vi "Edit Color List Dialog.vi"(10 "Color List":u32[](array[colorbox])=[16777225, 16448250, 16448250, 16448250, 16448250, 16448250, 16448250, 16448250, 16448250, 16448250], 11 "Color List Name":string) -> (0 "OK?":bool, 2 "Color List (out)":u32[](array[colorbox]), 3 "Color List Name (out)":string)   [LabVIEW 2019]
panel:
  in  "Cancel":bool
  in  "OK":bool
  out "# Colors":i32
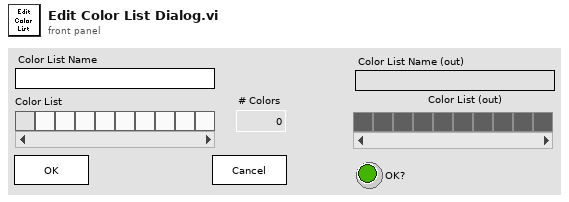
[diagram p1: front panel]
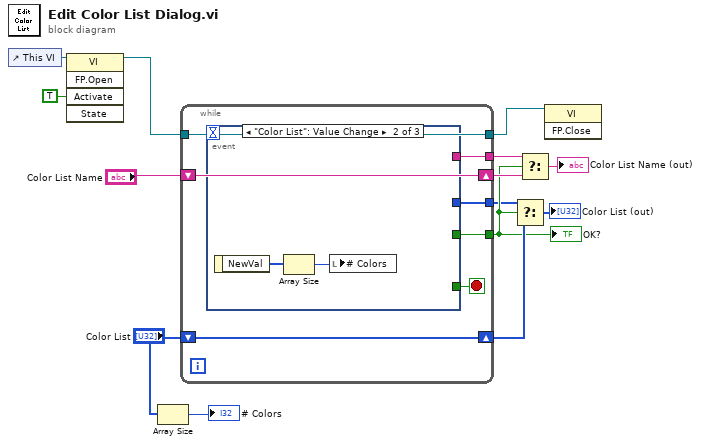
[diagram p0: block diagram]
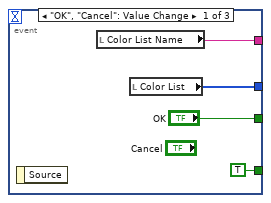
[diagram p2: hidden frame]
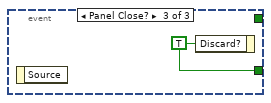
[diagram p3: hidden frame]
diagram:
  n1 = control-ref of="This VI"() -> (w14:refnum<vi>)
  n2 = invoke class="VI" method="FP.Open"(reference=w14, "Activate"=TRUE ("Activate?")) -> (reference out=w8:refnum<vi>)  [unwired: 3 in, 4 out]
  n3 = Array Size(array="Color List") -> (size(s)=→"# Colors":i32)
  n4 = while {
    tunnel: [w20] -> w3
    tunnel: w8 -> [w19]
    tunnel: [w19] -> w13
    shift-right: [w18] -> w12
    shift-left: "Color List" -> [w18]
    shift-right: [w17] -> w5
    shift-left: "Color List Name" -> [w17]
    tunnel: [w16] -> w2
    tunnel: [w15] -> w1
    stop <- w21 stop-if-true
    n5 = event shown="[1] \"Color List\": Value Change" {
      selector: _ -> [_ _ _]
      dyn-events: _ -> [_ _ _]
      timeout: _ -> [_ _ _]
      tunnel: [TRUE ("Discard?") _ w28] -> w21
      tunnel: ["OK" _ _] -> w20
      tunnel: [w23 _ _] -> w16
      tunnel: [w22 _ _] -> w15
      event "OK", "Cancel": Value Change {
        n6 = event-data() -> ()  [unwired: 1 in, 1 out]
        n7 = local read "Color List Name"() -> (w22:string)
        n8 = local read "Color List"() -> (w23:u32[])
      }
      event "Color List": Value Change {
        n9 = event-data() -> ("NewVal"=w27:u32[])  [unwired: 1 in]
        n10 = Array Size(array=w27) -> (size(s)=w26:i32)
        n11 = local write "# Colors"(w26) -> ()
      }
      event Panel Close? {
        w28 = TRUE ("Discard?")
        n12 = event-data() -> ()  [unwired: 1 in, 1 out]
        n13 = event-data("Discard?"=w28) -> ()  [unwired: 1 in, 1 out]
      }
    }
  }
  "OK?" <- w3
  n14 = Select(t=w2, s=w3, f=w12) -> (s? t:f=→"Color List (out)":u32[])
  n15 = Select(t=w1, s=w3, f=w5) -> (s? t:f=→"Color List Name (out)":string)
  n16 = invoke class="VI" method="FP.Close"(reference=w13) -> ()  [unwired: 2 in, 3 out]
